vi "PH_BL-Master.Release Objects from RC.vi"(0 "VI in":refnum<vi>, 5 "error in (no error)":errorcluster) -> (14 "VI out":refnum<vi>, 19 "error out":errorcluster)   [LabVIEW 2014, in "PH_BL-Master.lvlib"]
uses:
  PH_BL-Master.lvlib
  PH_Devices/PH_VacuumControl/PH_VacuumControl.lvlib
  PH_Basics/PH_Common/PH_Common.lvlib
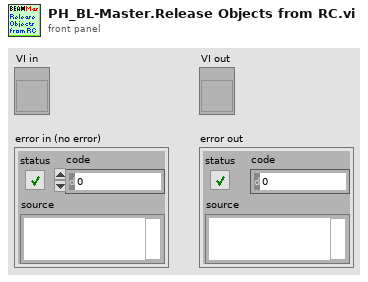
[diagram p1: front panel]
types:
  T1 = typedef "PH_BL-Master.lvlib/PH_BL-Master.i attribute.ctl" = cluster{"Remote controlled":bool, "Boolean Condition Service Subscriber":refnum<vi>[], "Picture Condition Service Subscriber":refnum<vi>[], "R2S":cluster{"GUI Ref":refnum<vi>, "State":bool}, "Vacua":cluster{"GUI Ref":refnum<vi>, "Limit":dbl, "Curr Value":dbl, "in range":bool}[], "O2 Inspection":cluster{"GUI Ref":refnum<vi>, "Concentration":dbl, "State":T2}[], "Boolean Status Service Subscriber":cluster{"GUI Ref":refnum<vi>, "Status":T2, "no Link?":bool, "Status Subscriber Class":T3}[], "Picture Status Service Subscriber":cluster{"GUI Ref":refnum<vi>, "Status":T2, "no Link?":bool, "Status Subscriber Class":T3}[], "6P 4Q Service Subscriber":cluster{"GUI Ref":refnum<vi>, "Selector":T4, "no Link?":bool}[], "Index of latest 6P 4Q changing Instance":i32, "Index of latest Picture Status changing Instance":i32, "Index of latest Boolean Status changing Instance":i32, "Vision ID on same Node":string, "Start Phase over?":bool, "GUI Ref Delete":refnum<vi>}
  T2 = typedef "PH_StatusHandler.lvlib/PH_StatusHandler.Status.ctl" = i16
  T3 = typedef "PH_BL-Master.lvlib/PH_BL-Master.Status Subscriber Class.ctl" = enum16{"unknown", "Switch", "BB", "6P Switch", "Switch GUI", "Switch and 6P State", "Force Sensor"}
  T4 = typedef "PH_4_Pos_Selector.lvlib/PH_4_Pos_Selector.Position Selector.ctl" = u16
  T5 = cluster{"GUI Ref":refnum<vi>, "Status":T2, "no Link?":bool, "Status Subscriber Class":T3}[]
  T6 = cluster{"GUI Ref":refnum<vi>, "Limit":dbl, "Curr Value":dbl, "in range":bool}[]
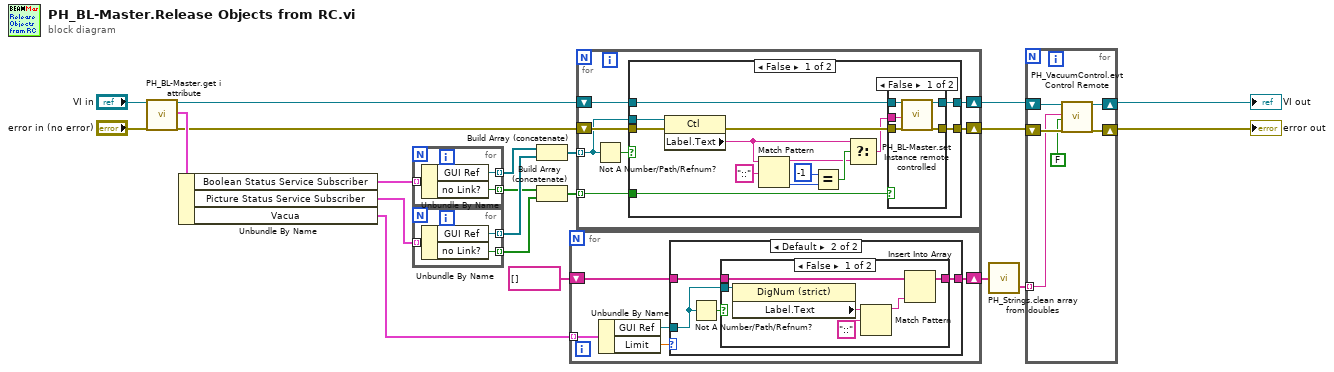
[diagram p0: block diagram]
diagram:
  n1 = call "PH_BL-Master.get i attribute.vi"("i ref in"="VI in", "error in (no error)"="error in (no error)") -> ("i ref out"=w13:refnum<vi>, "i attribute"=w16:T1, "error out"=w15:errorcluster)  [unwired: 15 in]
  n2 = Unbundle By Name(w16) -> ("Boolean Status Service Subscriber"=w3:T5, "Picture Status Service Subscriber"=w4:T5, "Vacua"=w9:T6)
  n3 = for {
    tunnel: w3 -> [w24] mode=indexing
    tunnel: [w23] -> w5 mode=indexing
    tunnel: [w22] -> w7 mode=indexing
    n4 = Unbundle By Name(w24) -> ("GUI Ref"=w23:refnum<vi>, "no Link?"=w22:bool)
  }
  n5 = for {
    tunnel: w4 -> [w27] mode=indexing
    tunnel: [w26] -> w8 mode=indexing
    tunnel: [w25] -> w6 mode=indexing
    n6 = Unbundle By Name(w27) -> ("GUI Ref"=w26:refnum<vi>, "no Link?"=w25:bool)
  }
  n7 = Build Array (concatenate)(w5, w8) -> (w10:refnum<vi>[])
  n8 = Build Array (concatenate)(w7, w6) -> (w11:bool[])
  n9 = for {
    tunnel: w9 -> [w32] mode=indexing
    shift-right: [w30] -> w19
    shift-left: string[] [] -> [w29]
    n10 = Unbundle By Name(w32) -> ("GUI Ref"=w31:refnum<vi>, "Limit"=w28:dbl)
    n11 = case shown="Default" w28 {
      tunnel: w31 -> [_ w36]
      tunnel: [w33 w35] -> w30
      tunnel: w29 -> [w33 w34]
      frame -1 {
      }
      frame Default {
        n12 = Not A Number/Path/Refnum?(number/path/refnum=w36) -> (NaN/Path/Refnum?=w37:bool)
        n13 = case shown="False" w37 {
          tunnel: w36 -> [w43 _]
          tunnel: [w40 w44] -> w35
          tunnel: w34 -> [w39 w44]
          frame False {
            n14 = property class="DigNum (strict)"(reference=w43) -> ("Label.Text"=w41:string)  [unwired: 1 in, 2 out]
            n15 = Match Pattern(string=w41, regular expression="::") -> (before substring=w38:string)  [unwired: 1 in, 3 out]
            n16 = Insert Into Array(array=w39, new element=w38) -> (w40:string[])  [unwired: 1 in]
          }
          frame True {
          }
        }
      }
    }
  }
  n17 = for {
    shift-right: [w49] -> w17
    shift-left: w13 -> [w50]
    shift-right: [w48] -> w18
    shift-left: w15 -> [w51]
    tunnel: w10 -> [w46] mode=indexing
    tunnel: w11 -> [w45] mode=indexing
    n18 = Not A Number/Path/Refnum?(number/path/refnum=w46) -> (NaN/Path/Refnum?=w47:bool)
    n19 = case shown="False" w47 {
      tunnel: w51 -> [w65 w73]
      tunnel: w50 -> [w64 w74]
      tunnel: [w63 w74] -> w49
      tunnel: [w62 w73] -> w48
      tunnel: w46 -> [w60 _]
      tunnel: w45 -> [w59 _]
      frame False {
        n20 = property class="Ctl"(reference=w60, error in=w65) -> (error out=w61:errorcluster, "Label.Text"=w54:string)  [unwired: 1 out]
        n21 = Match Pattern(string=w54, regular expression="::") -> (before substring=w52:string, offset past match=w57:i32)  [unwired: 1 in, 2 out]
        n22 = Equal?(x=-1, y=w57) -> (x = y?=w55:bool)
        n23 = Select(t=w54, s=w55, f=w52) -> (s? t:f=w53:string)
        n24 = case shown="False" w59 {
          tunnel: w61 -> [w70 w71]
          tunnel: w64 -> [w69 w72]
          tunnel: [w68 w72] -> w63
          tunnel: [w67 w71] -> w62
          tunnel: w53 -> [w66 _]
          frame False {
            n25 = call "PH_BL-Master.set Instance remote controlled.vi"("i ref in"=w69, "Instance Name"=w66, "error in"=w70) -> ("i ref out"=w68:refnum<vi>, "error out"=w67:errorcluster)  [unwired: 15 in]
          }
          frame True {
          }
        }
      }
      frame True {
      }
    }
  }
  n26 = call "PH_Strings.clean array from doubles.vi"("Array Input"=w19) -> ("Cleaned Array Output"=w21:string[])  [unwired: 1 out]
  n27 = for {
    shift-right: [w79] -> w1
    shift-left: w17 -> [w80]
    shift-right: [w77] -> w2
    shift-left: w18 -> [w78]
    tunnel: w21 -> [w76] mode=indexing
    n28 = call "PH_VacuumControl.evt Control Remote.vi"("i ref in"=w80, "Instance"=w76, "Control Remote?"=FALSE, "error in (no error)"=w78) -> ("i ref out"=w79:refnum<vi>, "error out"=w77:errorcluster)  [unwired: 14 in]
  }
  "error out" <- w2
  "VI out" <- w1
